vi "About.vi"() -> ()   [LabVIEW 2009]
doc: "This VI is used to illustrate the About box capability with LabVIEW executables."
panel:
  out "error out":errorcluster
  in  "error in (no error)":errorcluster
  # "LabVIEW Intermediate I\n\n\n\n\n\n\nCopyright ©2005 National Instruments Corporation.  All Rights Reserved."
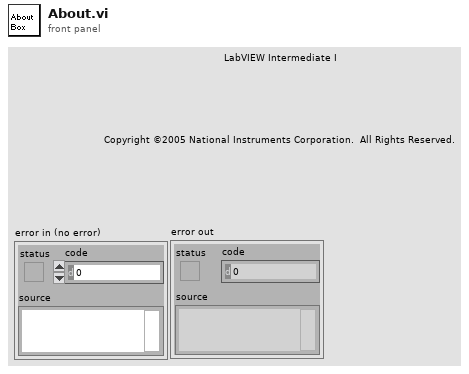
[diagram p1: front panel]
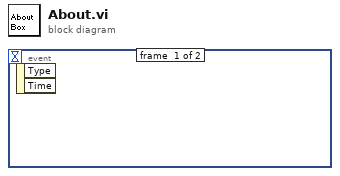
[diagram p0: block diagram]
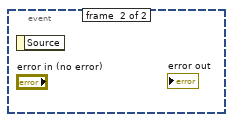
[diagram p2: hidden frame]
diagram:
  n1 = event shown="[1] \"Pane\": Mouse Down" {
    selector: _ -> [_ _]
    dyn-events: _ -> [_ _]
    timeout: _ -> [_ _]
    event #0 {
      n2 = event-data() -> ()  [unwired: 1 in, 2 out]
    }
    event #1 {
      n3 = event-data() -> ()  [unwired: 1 in, 1 out]
    }
  }
